vi "3-8 (Determine Warnings).vi"() -> ()   [LabVIEW 2014]
panel:
  out "Warning Text":string
  out "Warning?":bool
  in  "Min Temp":dbl
  in  "Max Temp":dbl
  in  "Current Temp":dbl
  # "You must create a portion of a larger project. The lead developer gives you the inputs of the VI, the\nalgorithm, and the expected outputs. Create and document a VI based on the given design."
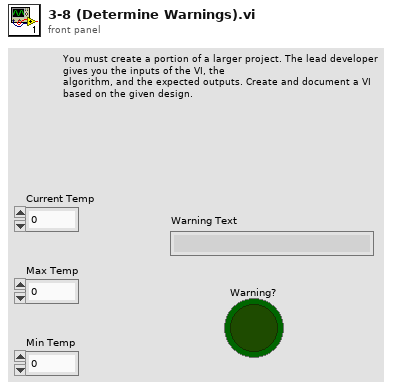
[diagram p1: front panel]
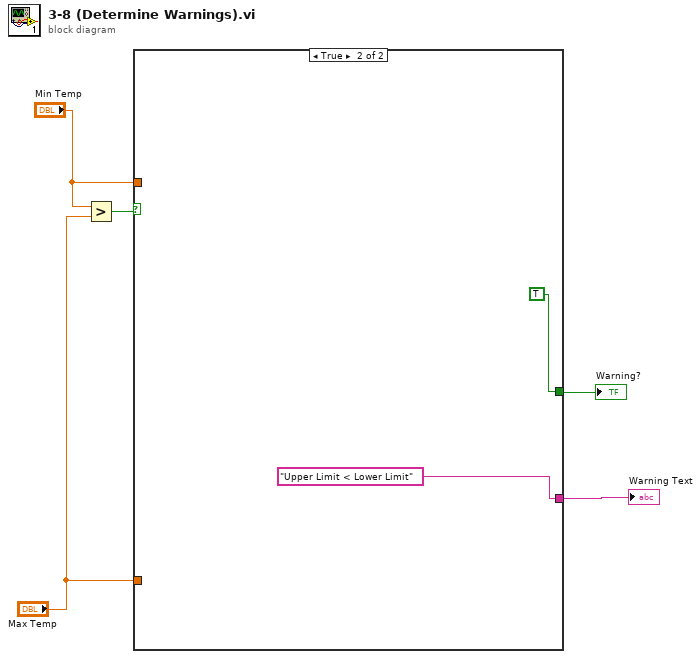
[diagram p0: block diagram]
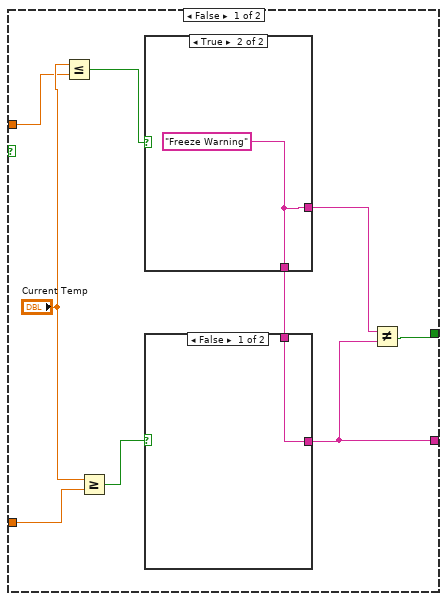
[diagram p2: hidden frame]
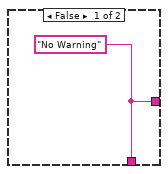
[diagram p3: hidden frame]
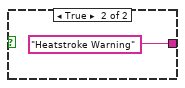
[diagram p4: hidden frame]
diagram:
  n1 = Greater?(x="Min Temp", y="Max Temp") -> (0:w2:bool)
  n2 = case shown="True" w2 {
    tunnel: [w13 TRUE] -> w5
    tunnel: "Max Temp" -> [w12 _]
    tunnel: "Min Temp" -> [w11 _]
    tunnel: [w6 "Upper Limit < Lower Limit"] -> w1
    frame False {
      n3 = Less Or Equal?(x="Current Temp", y=w11) -> (x <= y?=w9:bool)
      n4 = Greater Or Equal?(x="Current Temp", y=w12) -> (x >= y?=w10:bool)
      n5 = case shown="True" w9 {
        tunnel: [w15 w16] -> w8
        tunnel: [w15 w16] -> w7
        frame False {
          w15 = "No Warning"
        }
        frame True {
          w16 = "Freeze Warning"
        }
      }
      n6 = case shown="False" w10 {
        tunnel: [w17 "Heatstroke Warning"] -> w6
        tunnel: w8 -> [w17 _]
        frame False {
        }
        frame True {
        }
      }
      n7 = Not Equal?(x=w7, y=w6) -> (x != y?=w13:bool)
    }
    frame True {
    }
  }
  "Warning?" <- w5
  "Warning Text" <- w1
